vi "generate_config_2Chann_simultaneous_v2.vi"(0 "Generate config Chann1":T1={"maximum value"=5.0, "minimum value"=-5.0, "phase"=180.0, "amplitude"=1.0, "frequency"=10.0, "Wave Type"=0, "offset"=0.0} {"offset" format="%0.2p"; "Wave Type" items=["Sine", "Square", "Triangle", "Sawtooth", "DC Signal"]; "frequency" format="%0.2p"; "amplitude" format="%0.2p"}, 1 "Generate config Chann2":T1={"maximum value"=5.0, "minimum value"=-5.0, "phase"=180.0, "amplitude"=1.0, "frequency"=10.0, "Wave Type"=0, "offset"=0.0} {"offset" format="%0.2p"; "Wave Type" items=["Sine", "Square", "Triangle", "Sawtooth", "DC Signal"]; "frequency" format="%0.2p"; "amplitude" format="%0.2p"}) -> (2 "task out":refnum<k21>, 3 "signal Generated":waveform(dbl)[](graph), 4 "error out":errorcluster)   [LabVIEW 2017]
uses:
  <vilib>/DAQmx/write.llb/DAQmx Write (Analog 1D Wfm NChan NSamp).vi
  <vilib>/DAQmx/create/channels.llb/DAQmx Create Channel (AO-Voltage-Basic).vi
  <vilib>/DAQmx/configure/timing.llb/DAQmx Timing (Use Waveform).vi
  <vilib>/DAQmx/miscellaneous.llb/DAQmx Fill In Error Info.vi
  <instrlib>/NI USB-6356/NI USB-6356.lvlib
panel:
  in  "error in":errorcluster
  # "The lower freq. must be\nmultiple of the higher!!!"
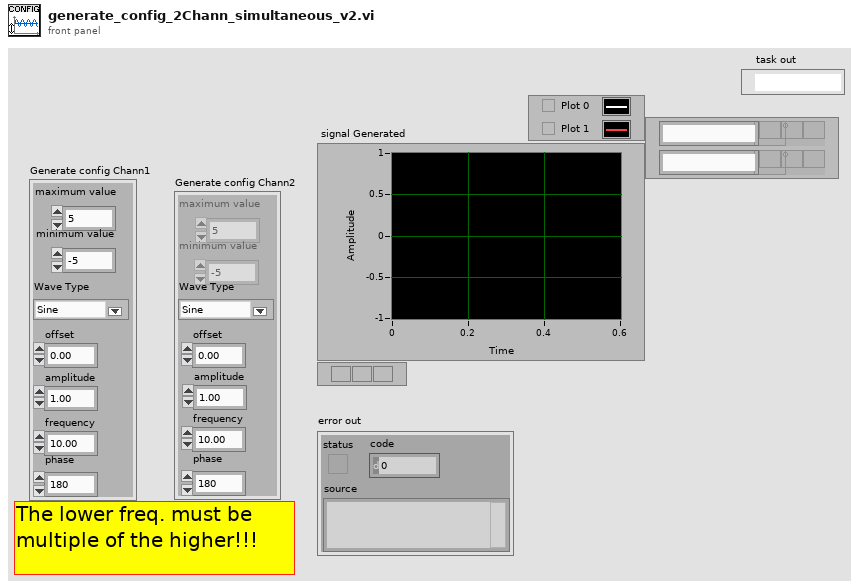
[diagram p1: front panel]
types:
  T1 = cluster{"maximum value":dbl, "minimum value":dbl, "phase":dbl, "amplitude":dbl, "frequency":dbl, "Wave Type":u16, "offset":dbl}
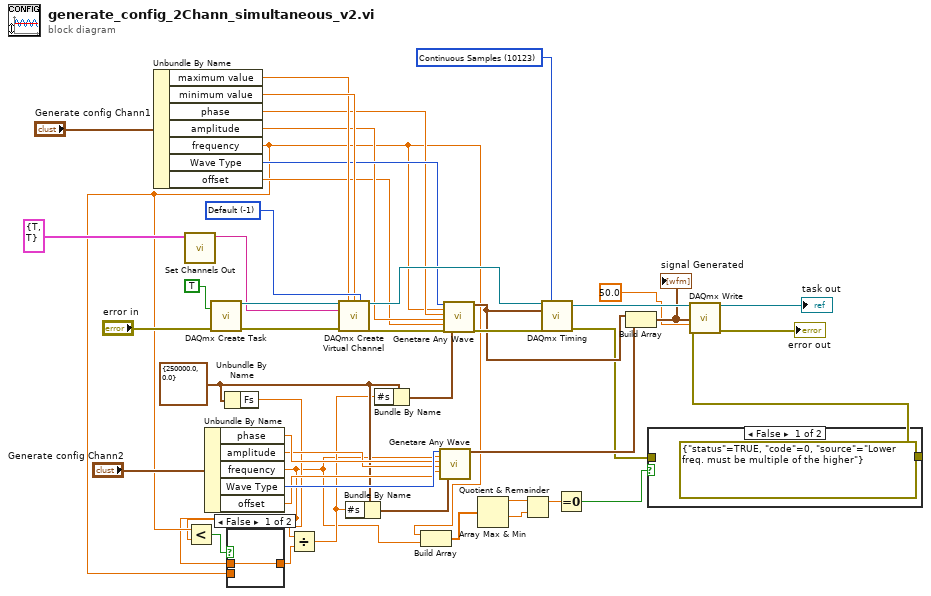
[diagram p0: block diagram]
diagram:
  w20 = cluster{"Fs":dbl, "#s":dbl} {"Fs"=250000.0, "#s"=0.0} ("sampling info 2")
  w43 = 10123 items=["Finite Samples"=10178, "Continuous Samples"=10123, "Hardware Timed Single Point"=12522] ("sample mode")
  w46 = -1 items=["Default"=-1, "RSE"=10083, "Differential"=10106, "Pseudodifferential"=12529] ("output terminal configuration")
  n1 = Unbundle By Name("Generate config Chann1") -> ("maximum value"=w35:dbl, "minimum value"=w36:dbl, "phase"=w31:dbl, "amplitude"=w30:dbl, "frequency"=w3:dbl, "Wave Type"=w32:u16, "offset"=w29:dbl)
  n2 = call <instrlib>:"Set Channels Out.vi"("Analog Out Channels"=cluster{"0":bool, "1":bool} {"0"=TRUE, "1"=TRUE}) -> ("String"=w33:string)  [unwired: 10 in]
  n3 = Unbundle By Name("Generate config Chann2") -> ("phase"=w25:dbl, "amplitude"=w24:dbl, "frequency"=w2:dbl, "Wave Type"=w26:u16, "offset"=w23:dbl)
  n4 = Less?(x=w3, y=w2) -> (x < y?=w19:bool)
  n5 = call <vilib>:"DAQmx Create Task.vi"("auto cleanup"=TRUE, "error in"="error in") -> ("task out"=w40:refnum<k21>, "error out"=w39:errorcluster)  [unwired: 12 in]
  n6 = Unbundle By Name(w20) -> ("Fs"=w10:dbl)
  n7 = case shown="False" w19 {
    tunnel: w2 -> [w47 _]
    tunnel: [w47 w48] -> w18
    tunnel: w3 -> [_ w48]
    frame False {
    }
    frame True {
    }
  }
  n8 = Divide(x=w10, y=w18) -> (x/y=w17:dbl)
  n9 = call-poly <vilib>:"DAQmx Create Virtual Channel.vi"("task in"=w40, "maximum value"=w35, "minimum value"=w36, "output terminal configuration"=w46, "physical channels"=w33, "error in"=w39) -> ("task out"=w45:refnum<k21>, "error out"=w28:errorcluster)  [unwired: 8 in]
  n10 = Bundle By Name(cluster=w20, "#s"=w17) -> (w21:cluster{"Fs":dbl, "#s":dbl})
  n11 = Bundle By Name(cluster=w20, "#s"=w17) -> (w22:cluster{"Fs":dbl, "#s":dbl})
  n12 = Build Array(w3, w2) -> (w1:dbl[])
  n13 = call <instrlib>:"Genetare Any Wave.vi"("Wave Type"=w26, "frequency"=w2, "phase"=w25, "amplitude"=w24, "Offset"=w23, "sampling info"=w21) -> ("Generated Signal 2"=w13:waveform(dbl))  [unwired: 12 in, 1 out]
  n14 = call <instrlib>:"Genetare Any Wave.vi"("Wave Type"=w32, "frequency"=w3, "phase"=w31, "amplitude"=w30, "Offset"=w29, "error in"=w28, "sampling info"=w22) -> ("Generated Signal 2"=w14:waveform(dbl), "error out"=w27:errorcluster)  [unwired: 11 in]
  n15 = Array Max & Min(array=w1) -> (max value=w5:dbl, min value=w4:dbl)  [unwired: 2 out]
  n16 = Quotient & Remainder(x=w5, y=w4) -> (x-y*floor(x/y)=w9:dbl)  [unwired: 1 out]
  n17 = call-poly <vilib>:"DAQmx Timing.vi"("task/channels in"=w45, "sample mode"=w43, "waveform"=w14, "error in"=w27) -> ("task out"=w44:refnum<k21>, "error out"=w8:errorcluster)  [unwired: 10 in]
  n18 = Equal To 0?(x=w9) -> (x = 0?=w6:bool)
  n19 = Build Array(w14, w13) -> (w12:waveform(dbl)[])
  "signal Generated" <- w12
  n20 = case shown="False" w6 {
    tunnel: [errorcluster {"status"=TRUE, "code"=0, "source"="Lower freq. must be multiple of the higher"} ("error out") w50] -> w7
    tunnel: w8 -> [_ w50]
    frame False {
    }
    frame True {
    }
  }
  n21 = call-poly <vilib>:"DAQmx Write.vi"("task/channels in"=w44, "data"=w12, "timeout"=50.0, "error in"=w7) -> ("task out"=→"task out":refnum<k21>, "error out"=→"error out":errorcluster)  [unwired: 9 in, 1 out]
